vi "Check Block Terminator.vi"(10 "Offset In":i32, 11 "Gif data in":string) -> (0 "Len":u8, 1 "Block Terminator?":bool, 2 "Offset Out":i32, 3 "Gif data Out":string)   [LabVIEW 2011, in "Gif Image.lvclass"]
uses:
  Gif Image.lvclass
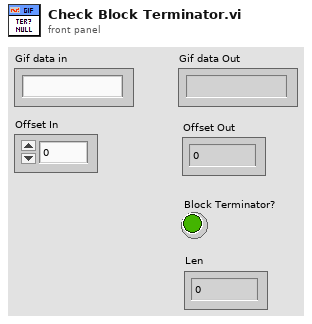
[diagram p1: front panel]
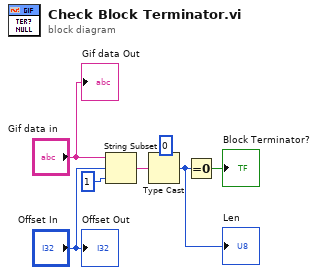
[diagram p0: block diagram]
diagram:
  n1 = String Subset(string="Gif data in", offset (0)="Offset In", length (rest)=1 ("长度（剩余）")) -> (substring=w4:string)
  n2 = Type Cast(type=u8 0, x=w4) -> (*(type *) &x=w1:u8)
  "Len" <- w1
  n3 = Equal To 0?(x=w1) -> (x = 0?=→"Block Terminator?":bool)
  "Offset Out" <- "Offset In"
  "Gif data Out" <- "Gif data in"
